vi "Convert To UV Map.vi"(7 "Texture Dimensions":T2, 11 "Point":T1) -> (3 "Point In Texture":T1)   [LabVIEW 2022 SP3, in "Raster.lvlib"]
uses:
  Raster.lvlib
  Point 2D.ctl
  Rectangle Dimensions.ctl
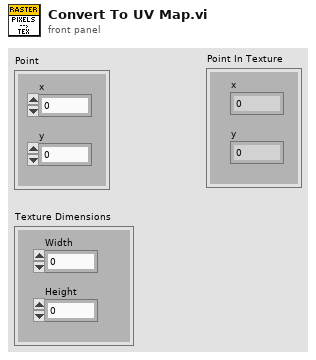
[diagram p1: front panel]
types:
  T1 = typedef "Raster.lvlib/Point 2D.ctl" = cluster{"x":i32, "y":i32}
  T2 = typedef "Raster.lvlib/Rectangle Dimensions.ctl" = cluster{"Width":u32, "Height":u32}
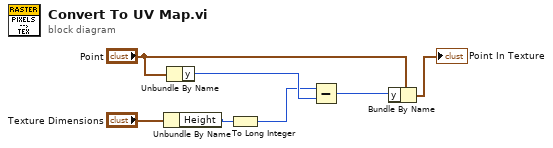
[diagram p0: block diagram]
diagram:
  n1 = Unbundle By Name("Texture Dimensions") -> ("Height"=w4:u32)
  n2 = Unbundle By Name("Point") -> ("y"=w3:i32)
  n3 = To Long Integer(number=w4) -> (32bit integer=w1:i32)
  n4 = Subtract(x=w1, y=w3) -> (x-y=w2:i32)
  n5 = Bundle By Name(cluster="Point", "y"=w2) -> (→"Point In Texture":T1)
